vi "Configure PLL.vi"(7 "instance":i32, 8 "error in":errorcluster, 10 "config":T1, 11 "lia host in":refnum<class "LIA Host Interface RT.lvclass">) -> (0 "error out":errorcluster, 3 "lia host out":refnum<class "LIA Host Interface RT.lvclass">)   [LabVIEW 2018, in "LIA Host Interface RT.lvclass"]
uses:
  LIA Host Interface RT.lvclass
  host/Public/pll settings.ctl
  shared/Public/message.ctl
  shared/Lock-In Amplifier Example Shared.lvlib
  host/Lock-In Amplifier Example Host.lvlib
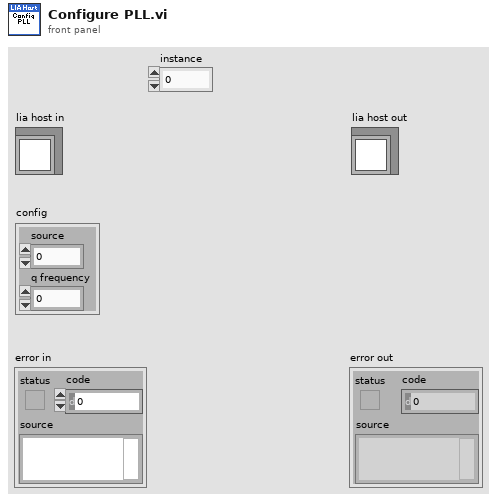
[diagram p1: front panel]
types:
  T1 = typedef "Lock-In Amplifier Example Host.lvlib/pll settings.ctl" = cluster{"source":i32, "q frequency":dbl}
  T2 = typedef "Lock-In Amplifier Example Shared.lvlib/message.ctl" = cluster{"command":u32, "payload":string}
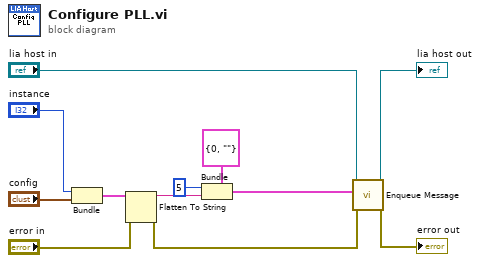
[diagram p0: block diagram]
diagram:
  n1 = Bundle("instance"="instance", "config"="config") -> (w12:cluster{"instance":i32, "config":T1})  [unwired: 1 in]
  n2 = Flatten To String(anything=w12, error in (no error)="error in") -> (data string=w11:string, error out=w8:errorcluster)  [unwired: 2 in, 1 out]
  n3 = Bundle(cluster=T2 {"command"=0, "payload"=""} ("message"), "command"=u32 5, "payload"=w11) -> (w10:T2)
  n4 = call "Enqueue Message.vi"("error in"=w8, "command"=w10, "lia host in"="lia host in") -> ("error out"=→"error out":errorcluster, "lia host out"=→"lia host out":refnum<class "LIA Host Interface RT.lvclass">)  [unwired: 7 in]
